vi "MonocromatorControl.vi"(2 "error in (no error)":errorcluster, 3 "Wavelength:":i16, 4 "ComPort:":refnum<visa-resource-name>="COM3") -> (0 "Error Out":errorcluster, 1 "return count":u32)   [LabVIEW 2014]
uses:
  <vilib>/Instr/_visa.llb/VISA Configure Serial Port (Instr).vi
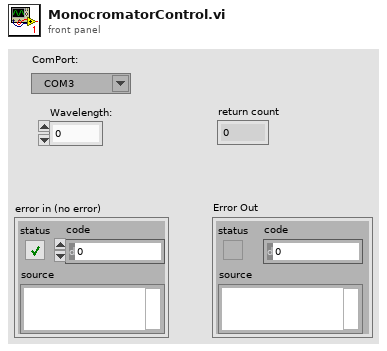
[diagram p1: front panel]
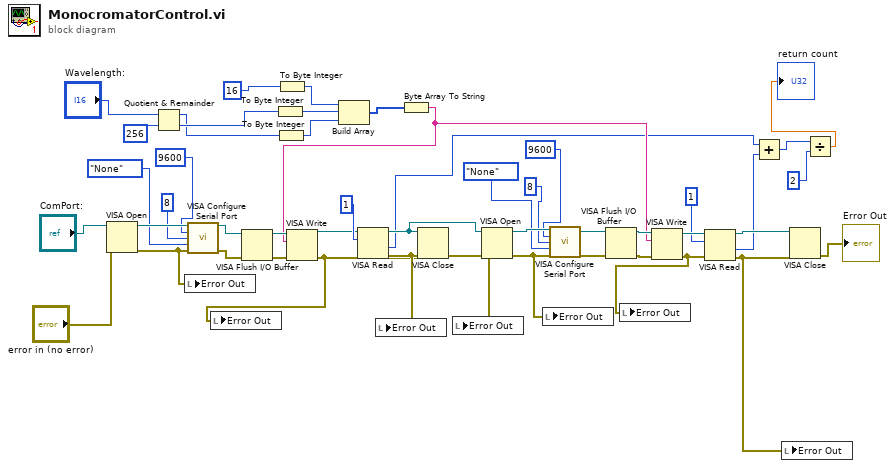
[diagram p0: block diagram]
diagram:
  n1 = VISA Open(error in (no error)="error in (no error)", VISA resource name="ComPort:") -> (VISA resource name=w45:refnum<visa-resource-name>, error out=w42:errorcluster)  [unwired: 3 in]
  n2 = Quotient & Remainder(x="Wavelength:", y=i16 256) -> (x-y*floor(x/y)=w28:i16, floor(x/y)=w29:i16)
  n3 = local write "Error Out"(w42) -> ()
  n4 = call-poly "VISA Configure Serial Port"("VISA resource name"=w45, "baud rate (9600)"=u32 9600, "data bits (8)"=u16 8, "parity (0:none)"=enum16{"None", "Odd", "Even", "Mark", "Space"}."None", "error in (no error)"=w42) -> ("VISA resource name out"=w44:refnum<visa-resource-name>, "error out"=w43:errorcluster)  [unwired: 9 in]
  n5 = VISA Flush I/O Buffer(VISA resource name=w44, error in (no error)=w43) -> (VISA resource name out=w46:refnum<visa-resource-name>, error out=w47:errorcluster)  [unwired: 1 in]
  n6 = To Byte Integer(number=w29) -> (8bit integer=w34:i8)
  n7 = To Byte Integer(number=w28) -> (8bit integer=w35:i8)
  n8 = To Byte Integer(number=u32 16) -> (8bit integer=w33:i8)
  n9 = Build Array(w33, w34, w35) -> (w32:i8[])
  n10 = Byte Array To String(unsigned byte array=w32) -> (string=w11:string)
  n11 = VISA Write(VISA resource name=w46, write buffer=w11, error in (no error)=w47) -> (VISA resource name out=w25:refnum<visa-resource-name>, error out=w24:errorcluster)  [unwired: 1 out]
  n12 = local write "Error Out"(w24) -> ()
  n13 = VISA Read(VISA resource name=w25, byte count=u32 1, error in (no error)=w24) -> (VISA resource name out=w14:refnum<visa-resource-name>, return count=w5:u32, error out=w27:errorcluster)  [unwired: 1 out]
  n14 = local write "Error Out"(w27) -> ()
  n15 = VISA Close(VISA resource name=w14, error in (no error)=w27) -> (error out=w15:errorcluster)
  n16 = local write "Error Out"(w15) -> ()
  n17 = VISA Open(error in (no error)=w15, VISA resource name=w14) -> (VISA resource name=w21:refnum<visa-resource-name>, error out=w9:errorcluster)  [unwired: 3 in]
  n18 = local write "Error Out"(w9) -> ()
  n19 = call-poly "VISA Configure Serial Port"("VISA resource name"=w21, "baud rate (9600)"=u32 9600, "data bits (8)"=u16 8, "parity (0:none)"=enum16{"None", "Odd", "Even", "Mark", "Space"}."None", "error in (no error)"=w9) -> ("VISA resource name out"=w20:refnum<visa-resource-name>, "error out"=w19:errorcluster)  [unwired: 9 in]
  n20 = VISA Flush I/O Buffer(VISA resource name=w20, error in (no error)=w19) -> (VISA resource name out=w22:refnum<visa-resource-name>, error out=w23:errorcluster)  [unwired: 1 in]
  n21 = VISA Write(VISA resource name=w22, write buffer=w11, error in (no error)=w23) -> (VISA resource name out=w16:refnum<visa-resource-name>, error out=w10:errorcluster)  [unwired: 1 out]
  n22 = local write "Error Out"(w10) -> ()
  n23 = VISA Read(VISA resource name=w16, byte count=u32 1, error in (no error)=w10) -> (VISA resource name out=w17:refnum<visa-resource-name>, return count=w4:u32, error out=w8:errorcluster)  [unwired: 1 out]
  n24 = Add(x=w5, y=w4) -> (x+y=w3:u32)
  n25 = local write "Error Out"(w8) -> ()
  n26 = VISA Close(VISA resource name=w17, error in (no error)=w8) -> (error out=→"Error Out":errorcluster)
  n27 = Divide(x=w3, y=u32 2) -> (x/y=→"return count":dbl)
